vi "Read Target.vi"(8 "error in (no error)":errorcluster, 11 "Power Supply in":refnum<class "Power Supply.lvclass">) -> (0 "error out":errorcluster, 2 "target":dbl[unit] caption="Target", 3 "Power Supply out":refnum<class "Power Supply.lvclass">)   [LabVIEW 2023, in "Power Supply.lvclass"]
uses:
  Power Supply.lvclass
  Power Supply.lvclass/Power Supply.ctl
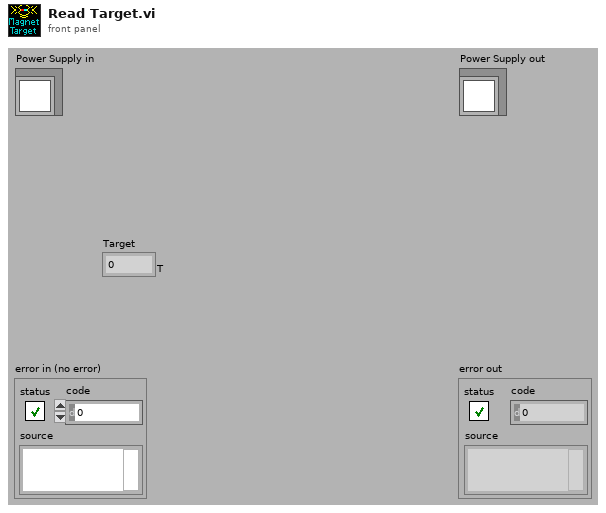
[diagram p1: front panel]
types:
  T1 = typedef "PSIO.ctl" = cluster{"Address":T2, "Version":enum16{"PS", "IPS"}}
  T2 = typedef "OxfordAddress.ctl" = cluster{"Com Port":i32, "ISOBUS Address":i32, "GPIB Address":i16, "Communication":enum16{"RS232", "ISOBUS", "GPIB", "Gateway"}}
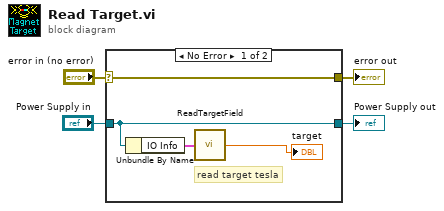
[diagram p0: block diagram]
diagram:
  n1 = case shown="No Error" "error in (no error)" {
    selector: "error in (no error)" -> [w8 w9]
    tunnel: [w8 w9] -> w3
    tunnel: [w7 w10] -> w2
    tunnel: "Power Supply in" -> [w7 w10]
    frame No Error {
      # "read target tesla"
      n2 = Unbundle By Name(w7) -> ("IO Info"=w6:T1)
      n3 = call "ReadTargetField.vi"("IO Info"=w6) -> ("Target field"=→"target":dbl[unit])  [unwired: 2 out]
    }
    frame Error {
    }
  }
  "error out" <- w3
  "Power Supply out" <- w2
